vi "GDSLvIcon_SplitString.vi"(2 "String":string, 5 "error in (no error)":errorcluster) -> (16 "words":string[](array[string]), 19 "error out":errorcluster)   [LabVIEW 2020]
doc: "Splits a string when ever a space, underscore or capital letter is found."
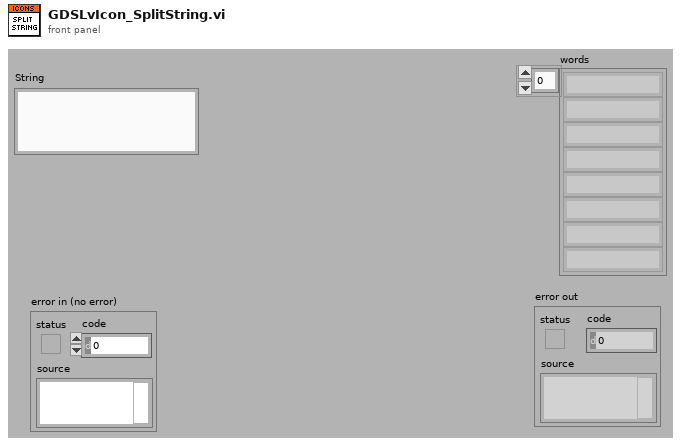
[diagram p1: front panel]
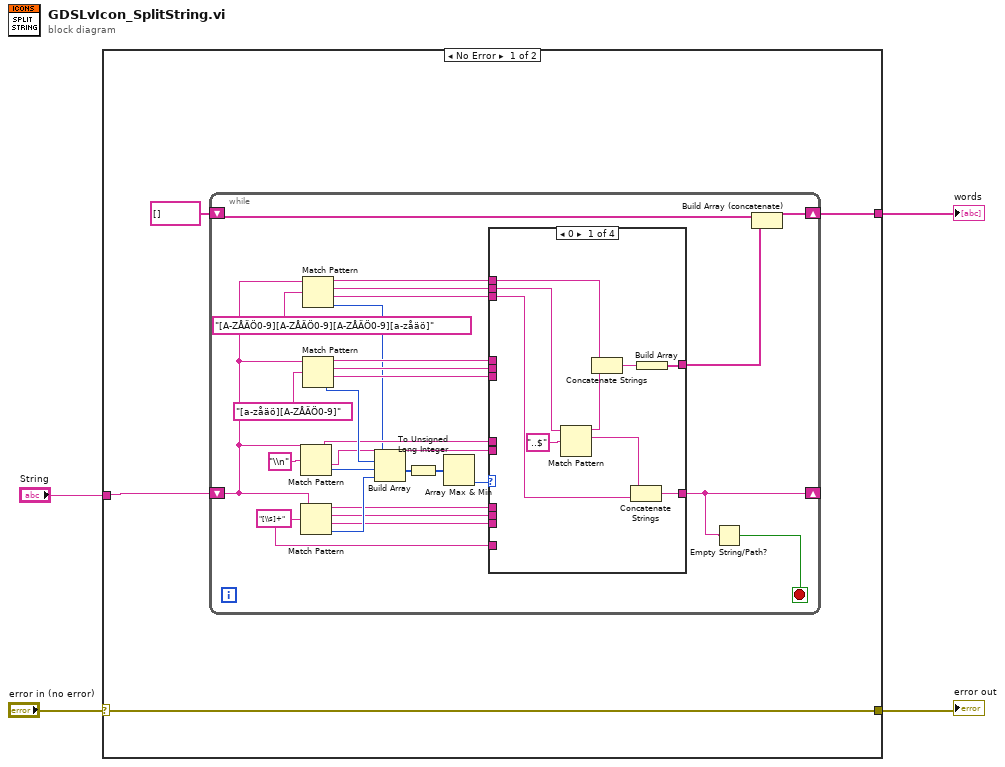
[diagram p0: block diagram]
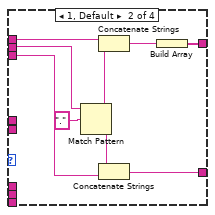
[diagram p2: hidden frame]
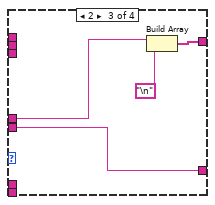
[diagram p3: hidden frame]
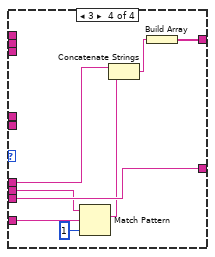
[diagram p4: hidden frame]
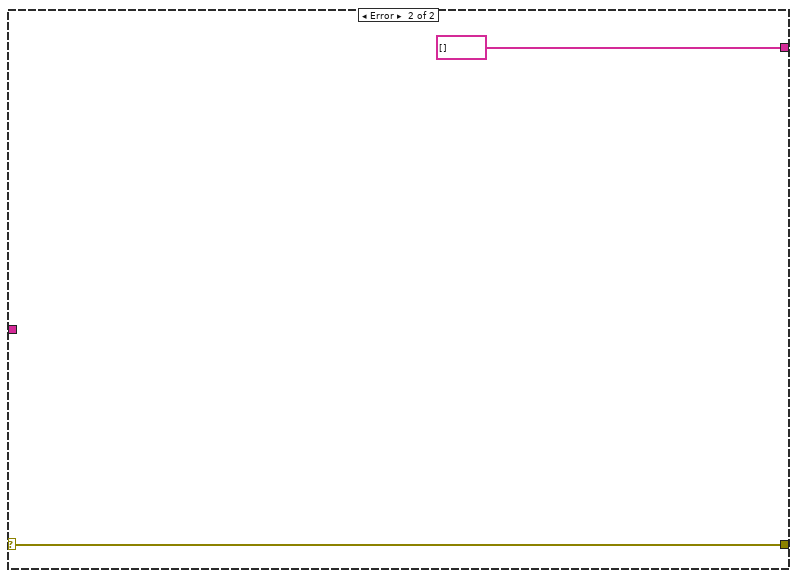
[diagram p5: hidden frame]
diagram:
  n1 = case shown="No Error" "error in (no error)" {
    selector: "error in (no error)" -> [w8 w68]
    tunnel: [w8 w68] -> w3
    tunnel: "String" -> [w6 _]
    tunnel: [w5 string[] [] ("Array Constant")] -> w1
    frame No Error {
      n2 = while {
        shift-left: string[] [] -> [w23]
        shift-right: [w22] -> w5
        shift-left: w6 -> [w12]
        shift-right: [w17] -> _
        stop <- w35 stop-if-true
        w36 = "[\\s]+" ("regular expression")
        n3 = Match Pattern(string=w12, regular expression="\\n") -> (before substring=w15:string, after substring=w20:string, offset past match=w31:i32)  [unwired: 1 in, 1 out]
        n4 = Match Pattern(string=w12, regular expression=w36) -> (before substring=w18:string, match substring=w16:string, after substring=w19:string, offset past match=w30:i32)  [unwired: 1 in]
        n5 = Match Pattern(string=w12, regular expression="[A-ZÅÄÖ0-9][A-ZÅÄÖ0-9][A-ZÅÄÖ0-9][a-zåäö]") -> (before substring=w9:string, match substring=w11:string, after substring=w10:string, offset past match=w14:i32)  [unwired: 1 in]
        n6 = Match Pattern(string=w12, regular expression="[a-zåäö][A-ZÅÄÖ0-9]") -> (before substring=w26:string, match substring=w25:string, after substring=w24:string, offset past match=w32:i32)  [unwired: 1 in]
        n7 = Build Array(w14, w32, w31, w30) -> (w29:i32[])
        n8 = To Unsigned Long Integer(number=w29) -> (unsigned 32bit integer=w28:u32[])
        n9 = Array Max & Min(array=w28) -> (min index (indices)=w27:i32)  [unwired: 3 out]
        n10 = case shown="0" w27 {
          tunnel: w26 -> [_ w54 _ _]
          tunnel: w25 -> [_ w52 _ _]
          tunnel: w24 -> [_ w53 _ _]
          tunnel: [w37 w48 w58 w66] -> w17
          tunnel: [w39 w46 w57 w59] -> w21
          tunnel: w20 -> [_ _ w58 _]
          tunnel: w19 -> [_ _ _ w66]
          tunnel: w18 -> [_ _ _ w62]
          tunnel: w16 -> [_ _ _ w65]
          tunnel: w36 -> [_ _ _ w63]
          tunnel: w15 -> [_ _ w56 _]
          tunnel: w11 -> [w43 _ _ _]
          tunnel: w10 -> [w41 _ _ _]
          tunnel: w9 -> [w40 _ _ _]
          frame 0 {
            n11 = Match Pattern(string=w43, regular expression="..$") -> (before substring=w38:string, match substring=w42:string)  [unwired: 1 in, 2 out]
            n12 = Concatenate Strings(w40, w38) -> (w44:string)
            n13 = Concatenate Strings(w42, w41) -> (w37:string)
            n14 = Build Array(w44) -> (w39:string[])
          }
          frame 1, Default {
            n15 = Match Pattern(string=w52, regular expression=".") -> (match substring=w50:string, after substring=w49:string)  [unwired: 1 in, 2 out]
            n16 = Concatenate Strings(w54, w50) -> (w47:string)
            n17 = Concatenate Strings(w49, w53) -> (w48:string)
            n18 = Build Array(w47) -> (w46:string[])
          }
          frame 2 {
            n19 = Build Array(w56, "\n") -> (w57:string[])
          }
          frame 3 {
            n20 = Match Pattern(string=w65, regular expression=w63, offset (0)=1) -> (match substring=w60:string)  [unwired: 3 out]
            n21 = Concatenate Strings(w62, w60) -> (w61:string)
            n22 = Build Array(w61) -> (w59:string[])
          }
        }
        n23 = Empty String/Path?(string/path=w17) -> (empty?=w35:bool)
        n24 = Build Array (concatenate)(w23, w21) -> (w22:string[])
      }
    }
    frame Error {
    }
  }
  "error out" <- w3
  "words" <- w1
